vi "GetSwerveAbsoluteAzimuth.vi"(1 "Relative Position (Raw Sensor Units)":i32) -> (0 "Azimuth Position (deg) [-180,+180]":dbl)   [LabVIEW 2019]
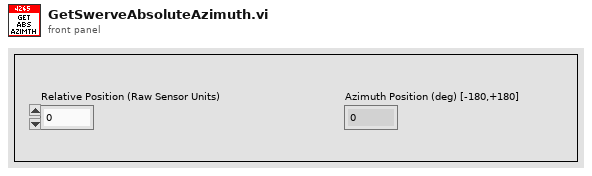
[diagram p1: front panel]
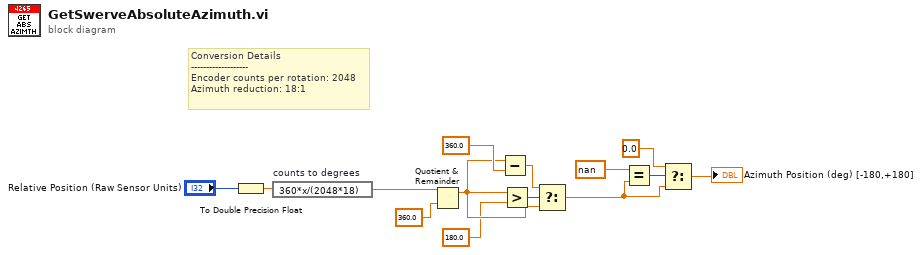
[diagram p0: block diagram]
diagram:
  # "Conversion Details\n-------------------\nEncoder counts per rotation: 2048\nAzimuth reduction: 18:1"
  n1 = To Double Precision Float(number="Relative Position (Raw Sensor Units)") -> (double precision float=w12:dbl)
  n2 = expression code="360*x/(2048*18)" "counts to degrees"(w12) -> (w14:dbl)
  n3 = Quotient & Remainder(x=w14, y=360.0) -> (x-y*floor(x/y)=w9:dbl)  [unwired: 1 out]
  n4 = Subtract(x=w9, y=360.0) -> (x-y=w10:dbl)
  n5 = Greater?(x=w9, y=180.0) -> (0:w8:bool)
  n6 = Select(t=w10, s=w8, f=w9) -> (s? t:f=w3:dbl)
  n7 = Equal?(x=nan, y=w3) -> (x = y?=w4:bool)
  n8 = Select(t=0.0, s=w4, f=w3) -> (s? t:f=→"Azimuth Position (deg) [-180,+180]":dbl)
